vi "number2-firewall logs.vi"() -> ()   [LabVIEW 2014]
uses:
  <vilib>/regexp/Match Regular Expression.xnode
panel:
  in  "Input String":string="Apr 26 21:31:34 filterlog: 129,16777216,,1425041642,hn0,match,pass,in,4,0x0,,128,16110,0,none,17,udp,36,10.2.10.175,255.255.255.255,60221,3956,16\nApr 26 21:31:34 filterlog: 129,16777216,,1425041642,hn0,match,pass,in,4,0x0,,128,4117,0,none,17,udp,78,10.2.10.1,208.93.4.206,137,137,58\nApr 26 21:31:32 filterlog: 130,16777216,,1425041643,hn0,match,pass,in,4,0x0,,128,18168,0,DF,17,udp,351,10.2.10.10,10.2.23.123,53,59118,331\nApr 26 21:31:32 filterlog: 129,16777216,,1425041642,hn0,match,pass,in,4,0x0,,128,10627,0,none,17,udp,82,10.2.10.10,140.112.2.2,59087,53,62\nApr 26 21:31:32 filterlog: 129,16777216,,1425041642,hn0,match,pass,in,4,0x0,,128,10626,0,none,17,udp,98,10.2.10.10,140.112.2.2,60847,53,78\nApr 26 21:38:10 filterlog: 105,16777216,,1425041627,hn1,match,block,in,4,0x2,0,109,9812,0,DF,6,tcp,48,207.46.13.171,10.2.10.15,25309,80,0,SEC,27892632,,8192,,mss;nop;nop;sackOK\nApr 26 21:38:08 filterlog: 129,16777216,,1425041642,hn0,match,pass,in,4,0x0,,128,23124,0,DF,6,tcp,52,10.2.10.172,207.46.153.155,60590,443,0,S,2141064781,,8192,,mss;nop;wscale;nop;nop;sackOK\nApr 26 21:38:08 filterlog: 130,16777216,,1425041643,hn0,match,block,in,4,0x2,0,128,8596,0,DF,6,tcp,48,10.2.10.2,10.2.102.10,41875,88,0,SEC,3256166066,,8192,,mss;nop;nop;sackOK\nApr 26 21:38:07 filterlog: 130,16777216,,1425041643,hn0,match,pass,in,4,0x2,0,128,8592,0,DF,6,tcp,48,10.2.10.2,10.2.102.10,41874,88,0,SEC,2184502132,,8192,,mss;nop;nop;sackOK"
  out "Array 2":string[][](array[string])
  out "array 2":string[](array[string])
  in  "stop running":bool
  out "array":string[](array[string])
  out "before substring":string
  in  "stop":bool
  out "Array":string[](array[string])
  # "Date-time            Interface-name            Protocol               Source-ip               Source-port             Target-ip                 Target-port                Length               Pass-or-block"
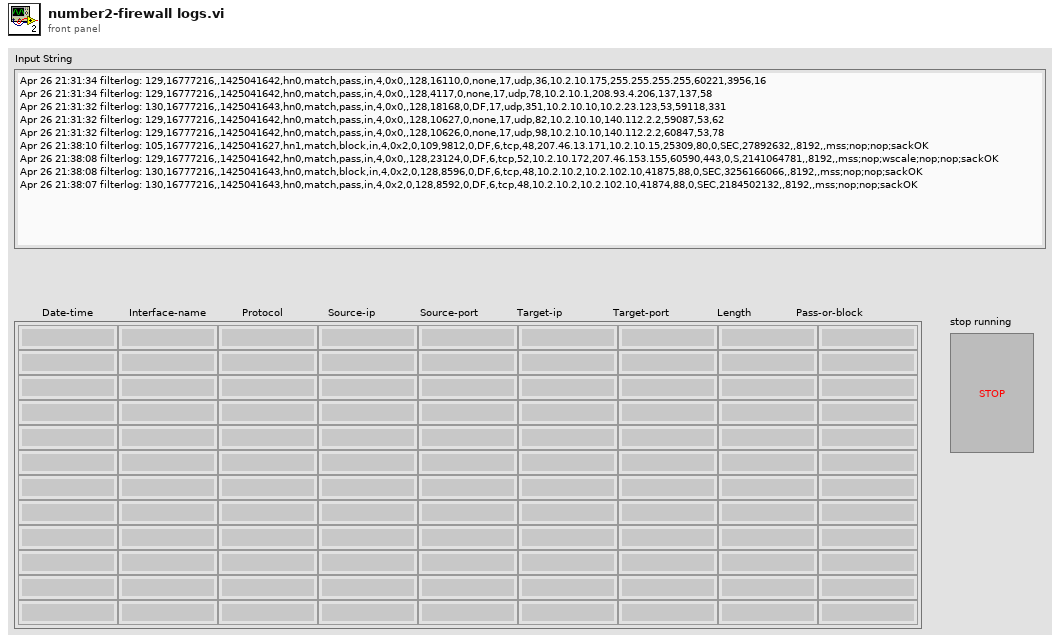
[diagram p1: front panel]
types:
  T1 = enum16{"open", "replace", "create", "open or create", "replace or create", "replace or create with confirmation"}
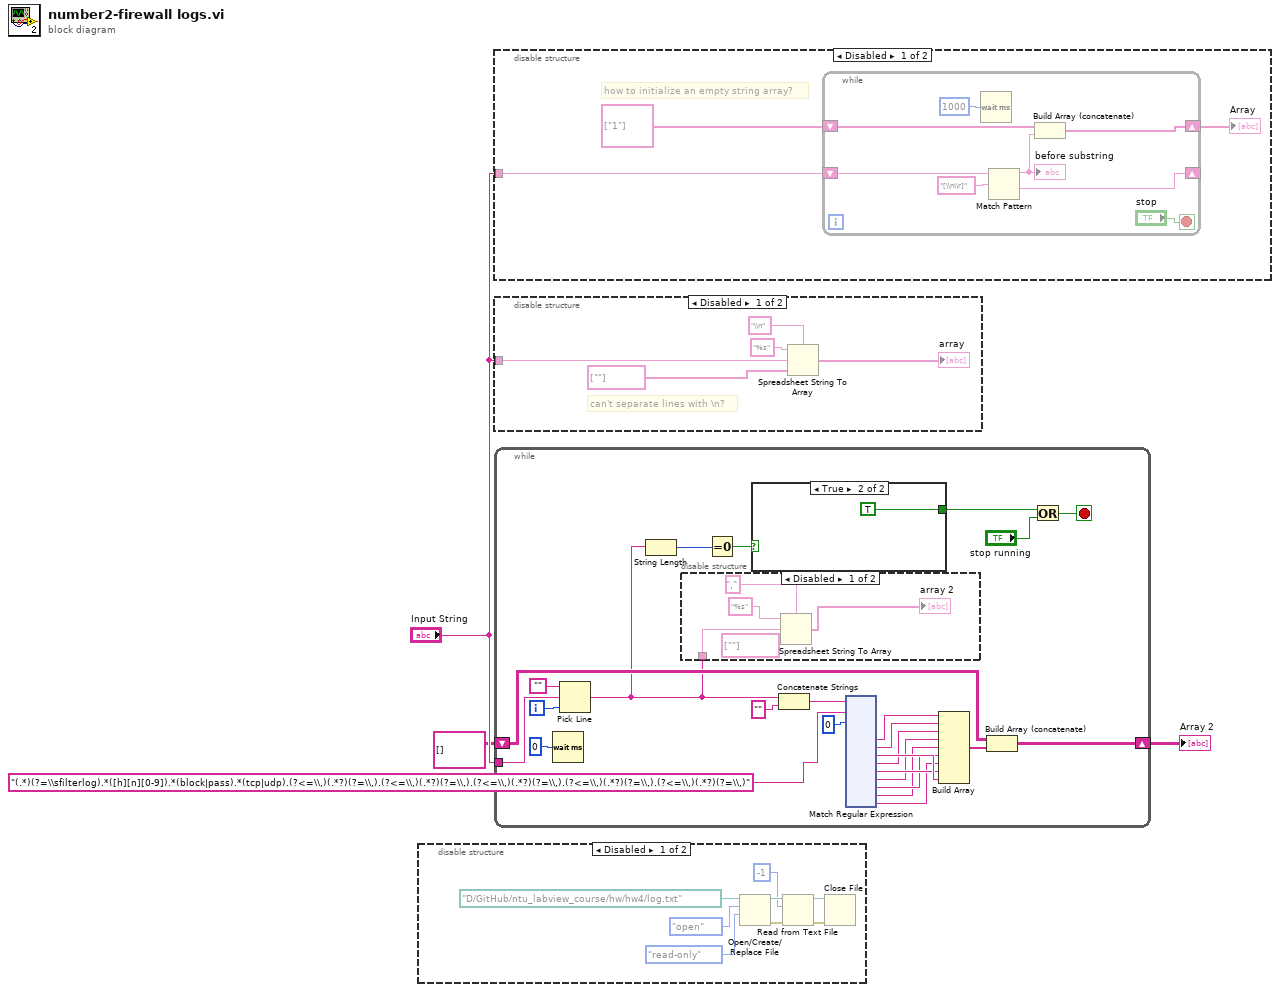
[diagram p0: block diagram]
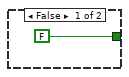
[diagram p5: hidden frame]
diagram:
  n1 = disable-structure shown="Disabled" {
    frame Disabled {
      n2 = Open/Create/Replace File(file path (use dialog)=path "D:/GitHub/ntu_labview_course/hw/hw4/log.txt", operation (0:open)=T1."open", access (0:read/write)=enum16{"read/write", "read-only", "write-only"}."read-only") -> (refnum out=w9:refnum<file>, error out=w7:errorcluster)  [unwired: 3 in, 1 out]
      n3 = Read from Text File(file (use dialog)=w9, count=-1, error in=w7) -> (refnum out=w8:refnum<file>, text=w4:string[], error out=w6:errorcluster)  [unwired: 1 in, 1 out]
      n4 = Close File(refnum=w8, error in=w6) -> ()  [unwired: 2 out]
    }
    frame Enabled {
    }
  }
  n5 = disable-structure shown="Disabled" {
    disable-tunnel: "Input String" -> [w13 _]
    frame Disabled {
      # "how to initialize an empty string array?"
      n6 = while {
        shift-right: [w21] -> _
        shift-left: w13 -> [w22]
        shift-right: [w18] -> w15
        shift-left: string[] ["1"] -> [w20]
        stop <- "stop" stop-if-true
        n7 = Wait (ms)(milliseconds to wait=u32 1000) -> ()  [unwired: 1 out]
        n8 = Match Pattern(string=w22, regular expression="[\\n\\r]") -> (before substring=w19:string, after substring=w21:string)  [unwired: 1 in, 2 out]
        "before substring" <- w19
        n9 = Build Array (concatenate)(w20, w19) -> (w18:string[])
      }
      "Array" <- w15
    }
    frame Enabled {
    }
  }
  n10 = disable-structure shown="Disabled" {
    disable-tunnel: "Input String" -> [w24 _]
    frame Disabled {
      # "can't separate lines with \\n?"
      n11 = Spreadsheet String To Array(delimiter (Tab)="\\n", format string="%s", spreadsheet string=w24, array type (2D Dbl)=string[] [""]) -> (array=→"array":string[])
    }
    frame Enabled {
    }
  }
  n12 = while {
    shift-right: [w44] -> w2
    shift-left: string[][] [] -> [w46]
    tunnel: "Input String" -> [w47]
    i -> [w54]
    stop <- w48 stop-if-true
    n13 = Wait (ms)(milliseconds to wait=u32 0) -> ()  [unwired: 1 out]
    n14 = Pick Line(string ("")="", multi-line string=w47, line index=w54) -> (output string=w40:string)
    n15 = String Length(string=w40) -> (length=w52:i32)
    n16 = disable-structure shown="Disabled" {
      disable-tunnel: w40 -> [w59 _]
      frame Disabled {
        n17 = Spreadsheet String To Array(delimiter (Tab)=",", format string="%s", spreadsheet string=w59, array type (2D Dbl)=string[] [""]) -> (array=→"array 2":string[])
      }
      frame Enabled {
      }
    }
    n18 = Equal To 0?(x=w52) -> (x = 0?=w51:bool)
    n19 = case shown="True" w51 {
      tunnel: [FALSE TRUE] -> w50
      frame False {
      }
      frame True {
      }
    }
    n20 = Concatenate Strings(w40, "" ("string")) -> (w43:string)
    n21 = xnode "Match Regular Expression"("input string"=w43, "regular expression"="(.*)(?=\\sfilterlog).*([h][n][0-9]).*(block|pass).*(tcp|udp).(?<=\\,)(.*?)(?=\\,).(?<=\\,)(.*?)(?=\\,).(?<=\\,)(.*?)(?=\\,).(?<=\\,)(.*?)(?=\\,).(?<=\\,)(.*?)(?=\\,)", "offset (0)"=0) -> ("submatch 1"=w38:string, "submatch 2"=w37:string, "submatch 3"=w36:string, "submatch 4"=w35:string, "submatch 5"=w34:string, "submatch 6"=w33:string, "submatch 7"=w32:string, "submatch 8"=w31:string, "submatch 9"=w30:string)  [unwired: 3 in, 5 out]
    n22 = Build Array(w38, w37, w35, w33, w31, w32, w30, w34, w36) -> (w39:string[])
    n23 = Build Array (concatenate)(w46, w39) -> (w44:string[][])
    n24 = Or(x=w50, y="stop running") -> (x .or. y?=w48:bool)
  }
  "Array 2" <- w2
